vi "Start Measurements.vi"(8 "error in (no error)":errorcluster, 9 "Repeat times":i32=1, 10 "Objects":string[](array[string]), 11 "Measure Controller in":refnum<class "Measure Controller.lvclass">) -> (0 "error out":errorcluster, 3 "Measure Controller out":refnum<class "Measure Controller.lvclass">)   [LabVIEW 2015, in "Measure Controller.lvclass"]
uses:
  Measure Controller.lvclass
  Measure Controller.lvclass/Measure Controller.ctl
  Measure Object/Measure Object.lvclass/Measure Object.ctl
  Measure Object/Write Repeat times.vi
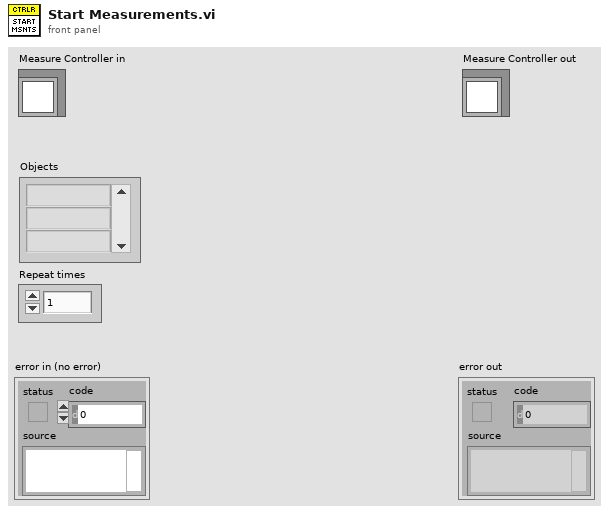
[diagram p1: front panel]
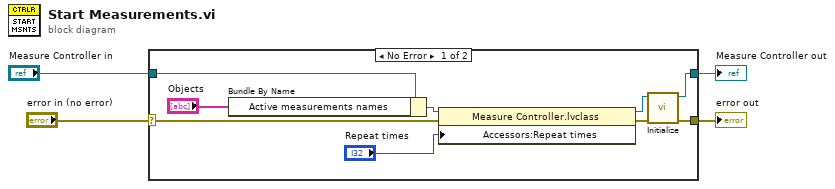
[diagram p0: block diagram]
diagram:
  n1 = case shown="No Error" "error in (no error)" {
    selector: "error in (no error)" -> [w6 w15]
    tunnel: [w5 w15] -> w3
    tunnel: [w10 w14] -> w1
    tunnel: "Measure Controller in" -> [w13 w14]
    frame No Error {
      n2 = Bundle By Name(cluster=w13, "Active measurements names"="Objects") -> (w11:refnum<class "Measure Controller.lvclass">)
      n3 = property class="Measure Controller.lvclass"(reference=w11, error in=w6, "Accessors:Repeat times"="Repeat times") -> (reference out=w9:refnum<class "Measure Controller.lvclass">, error out=w7:errorcluster)
      n4 = call-dynamic "Initialize.vi"("error in (no error)"=w7, "Measure Controller in"=w9) -> ("error out"=w5:errorcluster, "Measure Controller out"=w10:refnum<class "Measure Controller.lvclass">)  [unwired: 8 in]
    }
    frame Error {
    }
  }
  "error out" <- w3
  "Measure Controller out" <- w1
